vi "Write Old GoTo Params.vi"(8 "error in (no error)":errorcluster, 10 "Old GoTo Params":T1={"PID gains Angle GoTo"={"(Kc)"=3.0, "(Ki)"=0.0, "(Kd)"=2.0}, "PID gains XY GoTo"={"(Kc)"=3.0, "(Ki)"=0.0, "(Kd)"=2.0}, "Max Params GoTo"={"Max output XY"=3.0, "MaxOutput Angle"=0.0}}, 11 "Parameters in":refnum<class "Parameters.lvclass">) -> (0 "error out":errorcluster, 3 "Parameters out":refnum<class "Parameters.lvclass">)   [LabVIEW 2020, in "Parameters.lvclass"]
uses:
  Parameters.lvclass
  Parameters.lvclass/Parameters.ctl
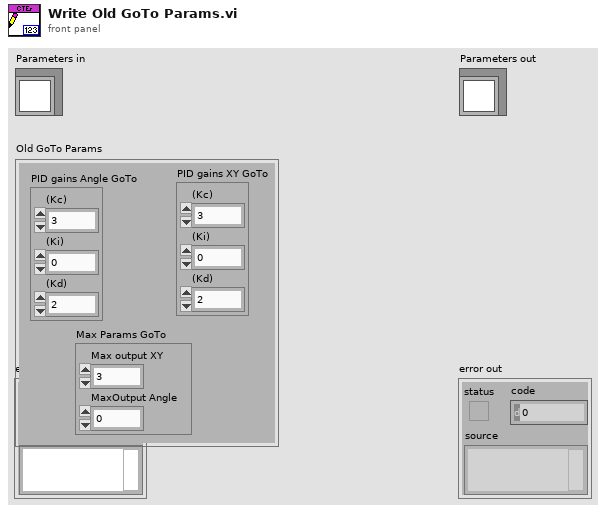
[diagram p1: front panel]
types:
  T1 = cluster{"PID gains Angle GoTo":cluster{"(Kc)":dbl, "(Ki)":dbl, "(Kd)":dbl}, "PID gains XY GoTo":cluster{"(Kc)":dbl, "(Ki)":dbl, "(Kd)":dbl}, "Max Params GoTo":cluster{"Max output XY":dbl, "MaxOutput Angle":dbl}}
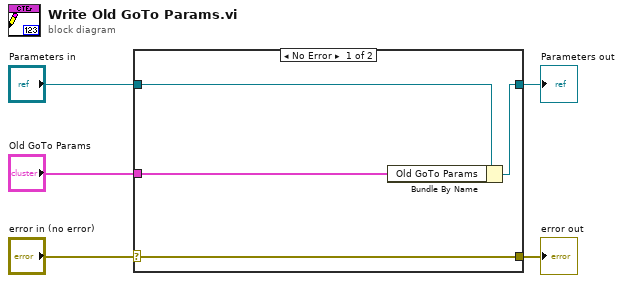
[diagram p0: block diagram]
diagram:
  n1 = case shown="No Error" "error in (no error)" {
    selector: "error in (no error)" -> [w9 w10]
    tunnel: [w9 w10] -> w4
    tunnel: [w7 w11] -> w2
    tunnel: "Parameters in" -> [w8 w11]
    tunnel: "Old GoTo Params" -> [w6 _]
    frame No Error {
      n2 = Bundle By Name(cluster=w8, "Old GoTo Params"=w6) -> (w7:refnum<class "Parameters.lvclass">)
    }
    frame Error {
    }
  }
  "error out" <- w4
  "Parameters out" <- w2
